vi "Font Family from File.vi"(8 "error in (no error)":errorcluster, 11 "Path":path) -> (0 "error out":errorcluster, 2 "FontCollection":refnum<k24>, 3 "Font":refnum<k24>)   [LabVIEW 2020, in "Glyph .NET.lvlib" / "Drawer .Net.lvclass"]
uses:
  Drawer .Net.lvclass
  System.Drawing
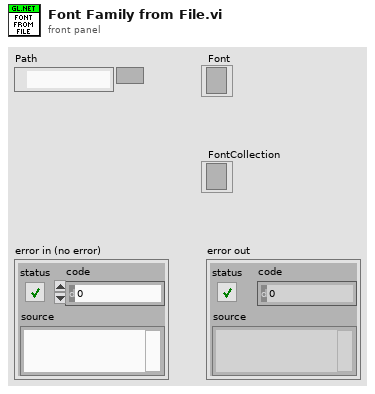
[diagram p1: front panel]
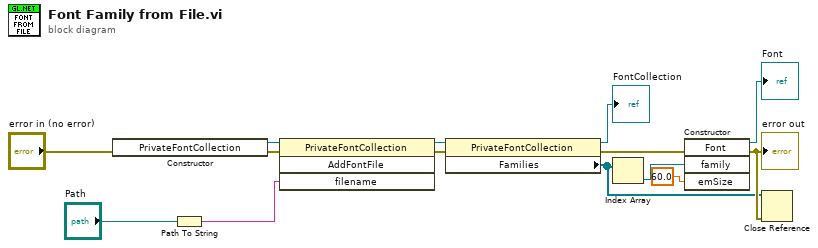
[diagram p0: block diagram]
diagram:
  n1 = constructor class="PrivateFontCollection"(error in="error in (no error)") -> (reference out=w11:refnum<k24>, error out=w9:errorcluster)  [unwired: 2 in, 1 out]
  n2 = Path To String(path="Path") -> (string=w12:string)
  n3 = invoke class="PrivateFontCollection" method="AddFontFile"(reference=w11, error in=w9, "filename"=w12) -> (reference out=w14:refnum<k24>, error out=w8:errorcluster)  [unwired: 1 in, 2 out]
  n4 = property class="PrivateFontCollection"(reference=w14, error in=w8) -> (reference out=→"FontCollection":refnum<k24>, error out=w6:errorcluster, "Families"=w1:refnum<k24>[])
  n5 = Index Array(array=w1) -> (element=w5:refnum<k24>)  [unwired: 1 in]
  n6 = constructor class="Font"(error in=w6, "family"=w5, "emSize"=sgl 60.0) -> (reference out=→"Font":refnum<k24>, error out=w2:errorcluster)  [unwired: 2 in, 3 out]
  "error out" <- w2
  n7 = Close Reference(reference=w1, error in (no error)=w2) -> ()  [unwired: 1 out]
